vi "get armed tracks.vi"(1 "Track Controls":T1 {"Track 3"."Volume" scale=0.01..10.0; "Track 3"."Pan" scale=0.0..1.0; "Track 2"."Volume" scale=0.01..10.0; "Track 2"."Pan" scale=0.0..1.0; "Track 1"."Volume" scale=0.01..10.0; "Track 1"."Pan" scale=0.0..1.0; "Track 0"."Volume" scale=0.01..10.0; "Track 0"."Pan" scale=0.0..1.0}) -> (0 "Track Enable":T3)   [LabVIEW 2014]
uses:
  Controls/Track Enable.ctl
  Controls/Track Controls.ctl
  Controls/Track Volume Settings.ctl
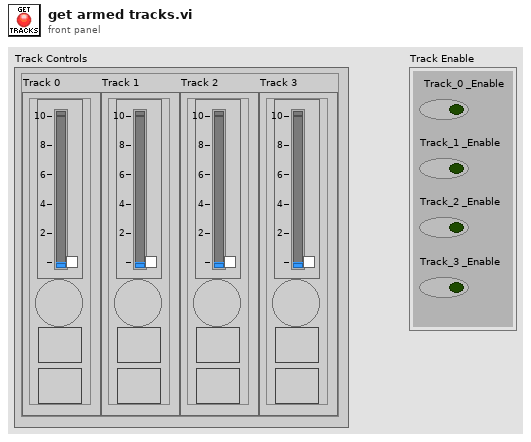
[diagram p1: front panel]
types:
  T1 = typedef "Track Controls.ctl" = cluster{"Track 0":T2, "Track 1":T2, "Track 2":T2, "Track 3":T2}
  T2 = typedef "Track Volume Settings.ctl" = cluster{"Volume":dbl, "Pan":dbl, "Record":bool, "FX":bool}
  T3 = typedef "Track Enable.ctl" = cluster{"Track_0 _Enable ":bool, "Track_1 _Enable ":bool, "Track_2 _Enable ":bool, "Track_3 _Enable ":bool}
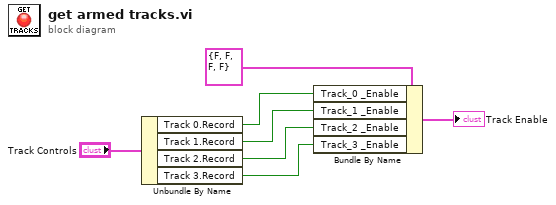
[diagram p0: block diagram]
diagram:
  n1 = Unbundle By Name("Track Controls") -> ("Track 0.Record"=w3:bool, "Track 1.Record"=w4:bool, "Track 2.Record"=w5:bool, "Track 3.Record"=w6:bool)
  n2 = Bundle By Name(cluster=T3 {"Track_0 _Enable "=FALSE, "Track_1 _Enable "=FALSE, "Track_2 _Enable "=FALSE, "Track_3 _Enable "=FALSE} ("Track Enable"), "Track_0 _Enable"=w3, "Track_1 _Enable"=w4, "Track_2 _Enable"=w5, "Track_3 _Enable"=w6) -> (→"Track Enable":T3)
